vi "ESN_DataPretreatment.vi"(8 "error in (no error)":errorcluster, 9 "Scale factor (2)":dbl=2.0, 10 "UserSettingsESN":T1, 11 "Data":dbl[][](array[numeric])) -> (0 "error out":errorcluster, 1 "output restore vector":dbl[](array[numeric]), 2 "input normalization vector":dbl[](array[numeric]), 3 "I/O pairs":cluster{dbl[], dbl[]}[](array[cluster]))   [LabVIEW 2017]
uses:
  UserSettingsESN.ctl
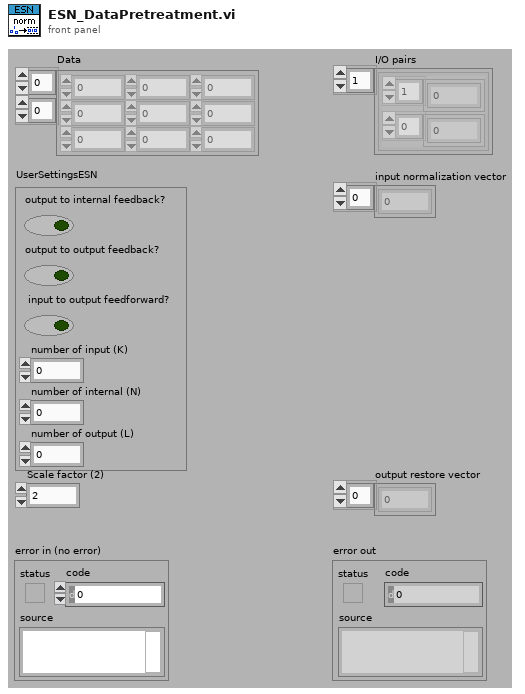
[diagram p1: front panel]
types:
  T1 = typedef "UserSettingsESN.ctl" = cluster{"output to internal feedback?":bool, "output to output feedback?":bool, " input to output feedforward?":bool, "number of input (K)":i32, "number of internal (N)":i32, "number of output (L)":i32}
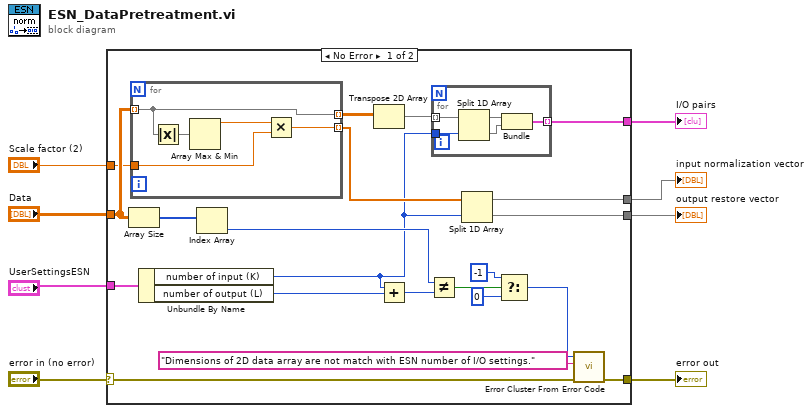
[diagram p0: block diagram]
diagram:
  n1 = case shown="No Error" "error in (no error)" {
    selector: "error in (no error)" -> [w11 w40]
    tunnel: "UserSettingsESN" -> [w29 _]
    tunnel: [w23 _] -> w7
    tunnel: "Data" -> [w21 _]
    tunnel: [w13 _] -> w5
    tunnel: [w12 _] -> w4
    tunnel: [w10 w40] -> w2
    tunnel: "Scale factor (2)" -> [w9 _]
    frame No Error {
      n2 = Array Size(array=w21) -> (size(s)=w28:i32[])
      n3 = for {
        tunnel: w21 -> [w31] mode=indexing
        tunnel: [w31] -> w20 mode=indexing
        tunnel: [w32] -> w15 mode=indexing
        tunnel: w9 -> [w30]
        n4 = Absolute Value(x=w31) -> (abs(x)=w33:dbl[])
        n5 = Array Max & Min(array=w33) -> (max value=w34:dbl)  [unwired: 3 out]
        n6 = Multiply(x=w34, y=w30) -> (x*y=w32:dbl)
      }
      n7 = Unbundle By Name(w29) -> ("number of input (K)"=w14:i32, "number of output (L)"=w26:i32)
      n8 = Index Array(array=w28) -> (element=w27:i32)  [unwired: 1 in]
      n9 = Transpose 2D Array(2D array=w20) -> (transposed array=w19:dbl[][])
      n10 = Add(x=w14, y=w26) -> (x+y=w25:i32)
      n11 = Not Equal?(x=w27, y=w25) -> (x != y?=w24:bool)
      n12 = for {
        tunnel: w19 -> [w39] mode=indexing
        tunnel: w14 -> [w38]
        tunnel: [w35] -> w23 mode=indexing
        n13 = Split 1D Array(array=w39, index=w38) -> (first subarray=w37:dbl[], second subarray=w36:dbl[])
        n14 = Bundle(w37, w36) -> (w35:cluster{dbl[], dbl[]})  [unwired: 1 in]
      }
      n15 = Split 1D Array(array=w15, index=w14) -> (first subarray=w13:dbl[], second subarray=w12:dbl[])
      n16 = Select(t=-1 ("number of input (K)"), s=w24, f=0) -> (s? t:f=w17:i32)
      n17 = call <vilib>:"Error Cluster From Error Code.vi"("error in (no error)"=w11, "error message (\"\")"="Dimensions of 2D data array are not match with ESN number of I/O settings." ("error message (\"\")"), "error code (0)"=w17) -> ("error out"=w10:errorcluster)  [unwired: 6 in]
    }
    frame Error {
    }
  }
  "I/O pairs" <- w7
  "input normalization vector" <- w5
  "output restore vector" <- w4
  "error out" <- w2
